vi "Actor Core.vi"(8 "error in":errorcluster, 11 "Save File in":refnum<class "Save File.lvclass">) -> (0 "error out":errorcluster, 3 "Actor out":refnum<class "Actor.lvclass">)   [LabVIEW 2018, in "Save File Actor.lvlib" / "Save File.lvclass"]
doc: "(<B>Filename</B>: Actor Framework.lvlib:Actor.lvclass:Actor Core.vi)\n\nReceives messages to the actor, reacts to them, and initiates any error handling that may shut the actor down.\n\nDescendant classes may override this VI to append parallel tasks for the actor to complete while it handles messages. Overrides use the Call Parent Method node."
uses:
  Save File.lvclass
  C:/Program Files (x86)/National Instruments/LabVIEW 2018/vi.lib/ActorFramework/Actor/Actor.lvclass
  <vilib>/ActorFramework/Actor/Actor.lvclass
  <vilib>/ActorFramework/Actor/Actor.lvclass/Actor.ctl
  <vilib>/ActorFramework/Message Enqueuer/Message Enqueuer.lvclass/Message Enqueuer.ctl
  Save File.lvclass/Save File.ctl
  <vilib>/ActorFramework/Message Enqueuer/Init from Existing Queue.vi
  <vilib>/ActorFramework/Message Enqueuer/Enqueue.vi
  <vilib>/ActorFramework/Stop Msg/Stop Msg.lvclass
  C:/Program Files (x86)/National Instruments/LabVIEW 2018/vi.lib/ActorFramework/Message/Message.lvclass
  <vilib>/ActorFramework/Message Priority Queue/Priority Enqueue.vi
  <vilib>/ActorFramework/Message Enqueuer/Message Enqueuer.lvclass
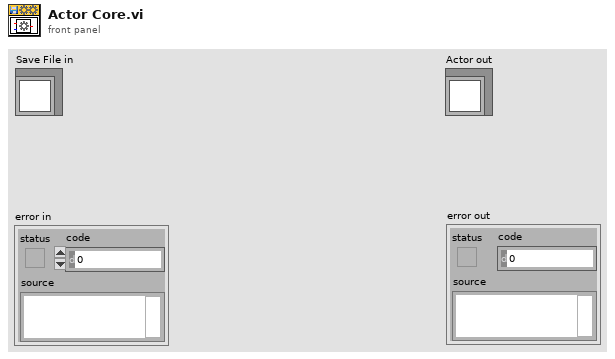
[diagram p1: front panel]
types:
  T1 = enum16{"open", "replace", "create", "open or create", "replace or create", "replace or create with confirmation"}
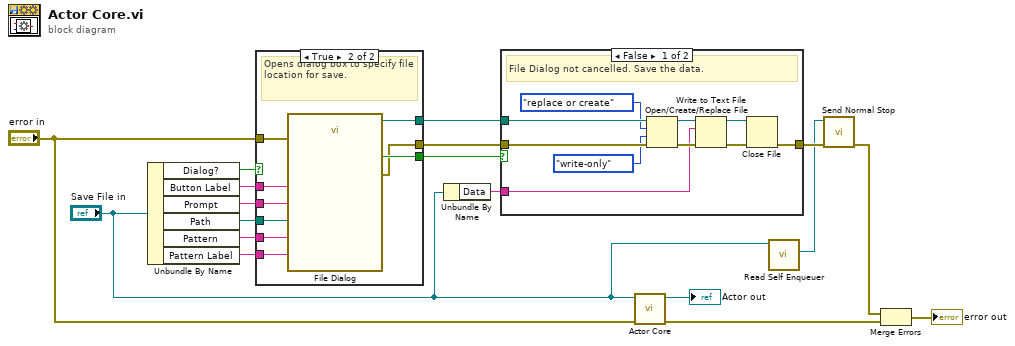
[diagram p0: block diagram]
diagram:
  n1 = Unbundle By Name("Save File in") -> ("Dialog?"=w16:bool, "Button Label"=w15:string, "Prompt"=w14:string, "Path"=w13:path, "Pattern"=w12:string, "Pattern Label"=w11:string)
  n2 = case shown="True" w16 {
    tunnel: w15 -> [_ w29]
    tunnel: w14 -> [_ w28]
    tunnel: w13 -> [w19 w27]
    tunnel: w12 -> [_ w26]
    tunnel: w11 -> [_ w25]
    tunnel: [_ w24] -> w9
    tunnel: [w19 w23] -> w8
    tunnel: "error in" -> [w20 w22]
    tunnel: [w20 w21] -> w7
    frame False {
      # "Passes the path through to save the file."
    }
    frame True {
      # "Opens dialog box to specify file location for save."
      n3 = call "File Dialog"("start path"=w27, "prompt"=w28, "button label"=w29, "error in"=w22, "pattern (all files)"=w26, "pattern label"=w25) -> ("selected path"=w23:path, "cancelled"=w24:bool, "error out"=w21:errorcluster)  [unwired: 6 in, 1 out]
    }
  }
  n4 = Unbundle By Name("Save File in") -> ("Data"=w6:string)
  n5 = case shown="False" w9 {
    tunnel: w8 -> [w39 _]
    tunnel: w7 -> [w38 w40]
    tunnel: w6 -> [w33 _]
    tunnel: [w30 w40] -> w2
    frame False {
      # "File Dialog not cancelled. Save the data."
      n6 = Open/Create/Replace File(file path (use dialog)=w39, error in=w38, operation (0:open)=T1."replace or create", access (0:read/write)=enum16{"read/write", "read-only", "write-only"}."write-only") -> (refnum out=w35:refnum<file>, error out=w34:errorcluster)  [unwired: 2 in, 1 out]
      n7 = Write to Text File(file (use dialog)=w35, text=w33, error in=w34) -> (refnum out=w31:refnum<file>, error out=w32:errorcluster)  [unwired: 1 in, 1 out]
      n8 = Close File(refnum=w31, error in=w32) -> (error out=w30:errorcluster)  [unwired: 1 out]
    }
    frame True {
      # "Do nothing if the File Dialog was cancelled."
    }
  }
  n9 = call-parent "Actor Core.vi"("error in"="error in", "Actor in"="Save File in") -> ("error out"=w18:errorcluster, "Actor out"=→"Actor out":refnum<class "Actor.lvclass">)  [unwired: 8 in]
  n10 = call <vilib>:"Read Self Enqueuer.vi"("Actor"="Save File in") -> ("Self Enqueuer"=w1:refnum<class "Message Enqueuer.lvclass">)  [unwired: 10 in]
  n11 = call <vilib>:"Send Normal Stop.vi"("error in (no error)"=w2, "Message Enqueuer"=w1) -> ("error out"=w3:errorcluster)  [unwired: 9 in]
  n12 = Merge Errors(w3, w18) -> (→"error out":errorcluster)
